vi "Set Detection.vi"(8 "error in (no error)":errorcluster, 9 "Optical Path":T1=1 items=["Eyepieces"=1, "Right"=2, "Bottom"=3, "Left"=4], 10 "Filter Position":T2=1 items=["1"=1, "2"=2, "3"=3, "4"=4, "5"=5, "6"=6], 11 "Virtual Microscope in":refnum<class "Virtual Microscope.lvclass">) -> (0 "error out":errorcluster, 3 "Virtual Microscope out":refnum<class "Virtual Microscope.lvclass">)   [LabVIEW 2018, in "Virtual Microscope.lvlib" / "Virtual Microscope.lvclass"]
uses:
  Virtual Microscope.lvclass
  Ti2/ti2lv/ti2_filterPos.ctl
  Ti2/ti2lv/ti2_lightPath.ctl
  Virtual Microscope.lvclass/Virtual Microscope.ctl
  Ti2 Messages/Set Detection Msg/Set Detection Msg.lvclass/Set Detection Msg.ctl
  <vilib>/ActorFramework/Message Enqueuer/Message Enqueuer.lvclass/Message Enqueuer.ctl
  <vilib>/ActorFramework/Message Enqueuer/Enqueue.vi
  Ti2 Messages/Set Detection Msg/Set Detection Msg.lvclass
  C:/Program Files/National Instruments/LabVIEW 2018/vi.lib/ActorFramework/Message/Message.lvclass
  <vilib>/ActorFramework/Message Priority Queue/Priority Enqueue.vi
  Ti2/ti2lv/ti2lv.lvlib
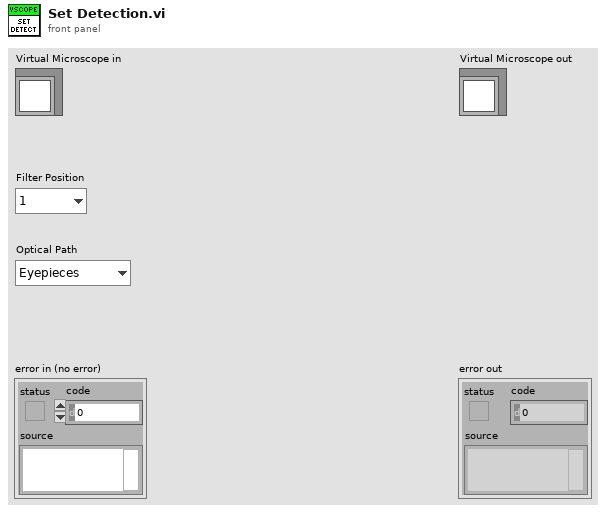
[diagram p1: front panel]
types:
  T1 = typedef "ti2lv.lvlib/ti2_lightPath.ctl" = i32
  T2 = typedef "ti2lv.lvlib/ti2_filterPos.ctl" = u16
  T3 = typedef "Microscope Type.ctl" = enum16{"Disable", "TE2000", "Eclipse Ti", "Ti2"}
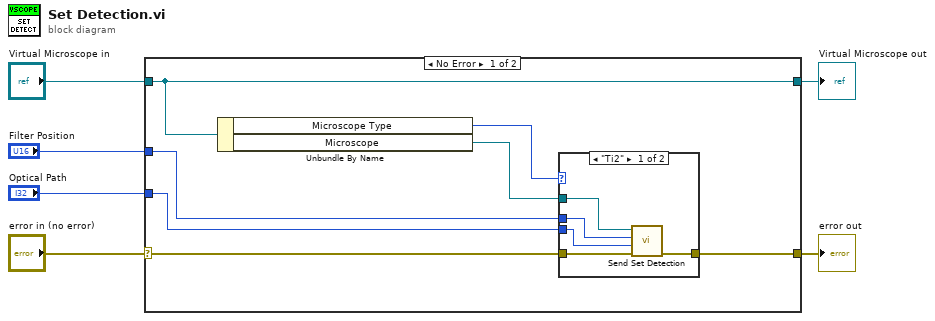
[diagram p0: block diagram]
diagram:
  n1 = case shown="No Error" "error in (no error)" {
    selector: "error in (no error)" -> [w12 w21]
    tunnel: [w11 w21] -> w5
    tunnel: [w9 w20] -> w3
    tunnel: "Virtual Microscope in" -> [w9 w20]
    tunnel: "Filter Position" -> [w10 _]
    tunnel: "Optical Path" -> [w7 _]
    frame No Error {
      n2 = Unbundle By Name(w9) -> ("Microscope Type"=w13:T3, "Microscope"=w8:refnum<class "Message Enqueuer.lvclass">)
      n3 = case shown="\"Ti2\"" w13 {
        tunnel: w8 -> [w18 _]
        tunnel: w12 -> [w17 w19]
        tunnel: [w16 w19] -> w11
        tunnel: w10 -> [w14 _]
        tunnel: w7 -> [w15 _]
        frame "Ti2" {
          n4 = call "Send Set Detection.vi"("error in (no error)"=w17, "Optical Path"=w15, "Filter Position"=w14, "Message Enqueuer"=w18) -> ("error out"=w16:errorcluster)  [unwired: 6 in, 1 out]
        }
        frame "Disable", Default {
        }
      }
    }
    frame Error {
    }
  }
  "error out" <- w5
  "Virtual Microscope out" <- w3
